vi "Check data length.vi"(11 "# samples in buffer":u16) -> (2 "Modbus Function":T1, 3 "# samples in buffer out":u16)   [LabVIEW 2017]
uses:
  Modbus function.ctl
panel:
  in  "bulk mode trigger (size)":u16=1230
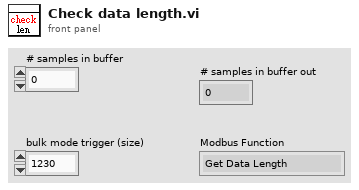
[diagram p1: front panel]
types:
  T1 = typedef "Modbus function.ctl" = enum16{"Get Data Length", "Normal Mode", "Bulk Mode"}
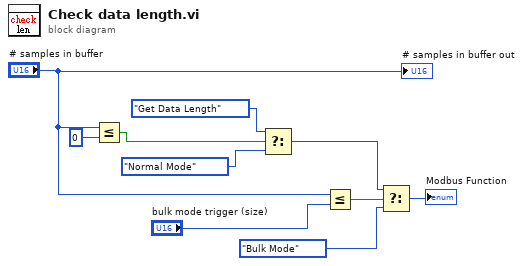
[diagram p0: block diagram]
diagram:
  n1 = Less Or Equal?(x="# samples in buffer", y=u16 0) -> (x <= y?=w9:bool)
  n2 = Select(t=Modbus_function."Get Data Length" ("Modbus"), s=w9, f=Modbus_function."Normal Mode" ("Modbus")) -> (s? t:f=w6:T1)
  n3 = Less Or Equal?(x="# samples in buffer", y="bulk mode trigger (size)") -> (x <= y?=w7:bool)
  n4 = Select(t=w6, s=w7, f=Modbus_function."Bulk Mode" ("Modbus")) -> (s? t:f=→"Modbus Function":T1)
  "# samples in buffer out" <- "# samples in buffer"
